vi "gaussmeter zero probes.vi"(8 "error in (no error)":errorcluster, 11 "VISA resource name":refnum<visa-resource-name>="GPIB1::11::INSTR") -> (0 "error out":errorcluster, 3 "VISA resource name":refnum<visa-resource-name>)   [LabVIEW 2013]
panel:
  # "This .vi calibrates the three Hall probes to 0T. It takes 1.25 min. to complete."
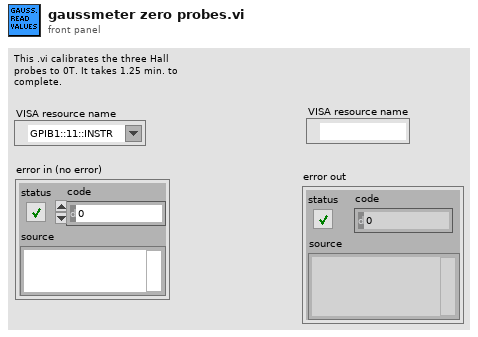
[diagram p1: front panel]
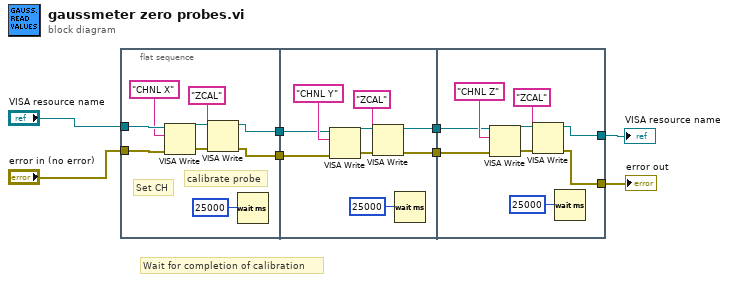
[diagram p0: block diagram]
diagram:
  # "Wait for completion of calibration"
  n1 = flat-sequence {
    tunnel: "VISA resource name" -> [w17]
    tunnel: "error in (no error)" -> [w16]
    tunnel: [w10] -> w6
    tunnel: [w9] -> w3
    tunnel: w6 -> [w21]
    tunnel: [w20] -> w5
    tunnel: w3 -> [w19]
    tunnel: [w18] -> w2
    tunnel: w5 -> [w30]
    tunnel: [w29] -> w4
    tunnel: w2 -> [w28]
    tunnel: [w27] -> w1
    frame #0 {
      # "calibrate probe"
      # "Set CH"
      n2 = VISA Write(VISA resource name=w17, write buffer="CHNL X", error in (no error)=w16) -> (VISA resource name out=w13:refnum<visa-resource-name>, error out=w14:errorcluster)  [unwired: 1 out]
      n3 = VISA Write(VISA resource name=w13, write buffer="ZCAL", error in (no error)=w14) -> (VISA resource name out=w10:refnum<visa-resource-name>, error out=w9:errorcluster)  [unwired: 1 out]
      n4 = Wait (ms)(milliseconds to wait=25000) -> ()  [unwired: 1 out]
    }
    frame #1 {
      n5 = VISA Write(VISA resource name=w21, write buffer="CHNL Y", error in (no error)=w19) -> (VISA resource name out=w24:refnum<visa-resource-name>, error out=w25:errorcluster)  [unwired: 1 out]
      n6 = VISA Write(VISA resource name=w24, write buffer="ZCAL", error in (no error)=w25) -> (VISA resource name out=w20:refnum<visa-resource-name>, error out=w18:errorcluster)  [unwired: 1 out]
      n7 = Wait (ms)(milliseconds to wait=25000) -> ()  [unwired: 1 out]
    }
    frame #2 {
      n8 = VISA Write(VISA resource name=w30, write buffer="CHNL Z", error in (no error)=w28) -> (VISA resource name out=w33:refnum<visa-resource-name>, error out=w34:errorcluster)  [unwired: 1 out]
      n9 = VISA Write(VISA resource name=w33, write buffer="ZCAL", error in (no error)=w34) -> (VISA resource name out=w29:refnum<visa-resource-name>, error out=w27:errorcluster)  [unwired: 1 out]
      n10 = Wait (ms)(milliseconds to wait=25000) -> ()  [unwired: 1 out]
    }
  }
  "VISA resource name" <- w4
  "error out" <- w1
